vi "RTM - Export to XML.vi"(8 "error in (no error)":errorcluster, 11 "Node Ptr":u64 format="%.0x") -> (0 "error out":errorcluster)   [LabVIEW 2019, in "UDP-Custom-Device System Explorer.lvlib"]
uses:
  UDP-Custom-Device System Explorer.lvlib
panel:
  in  "Tag":string
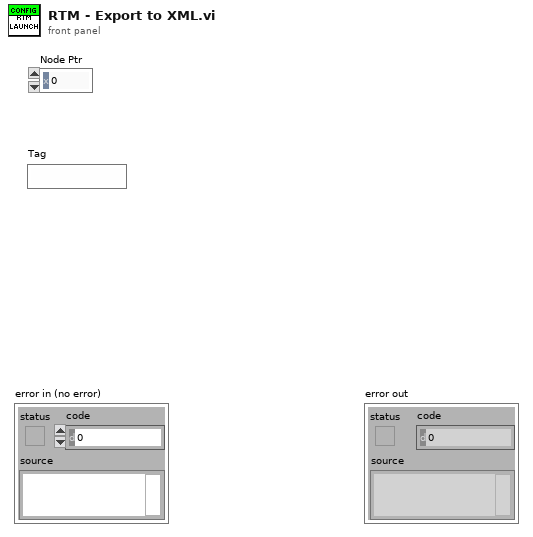
[diagram p1: front panel]
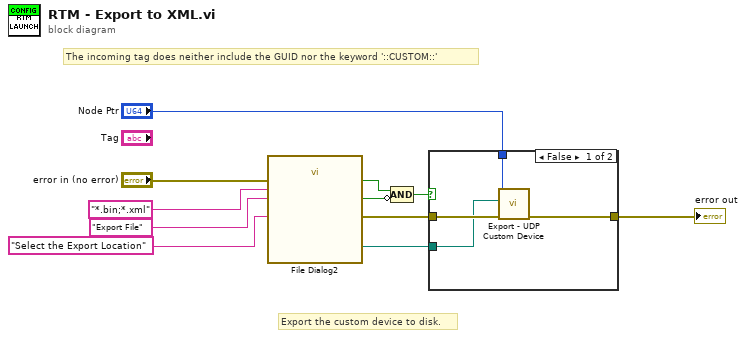
[diagram p0: block diagram]
diagram:
  # "Export the custom device to disk."
  # "The incoming tag does neither include the GUID nor the keyword '::CUSTOM::'"
  n1 = call "File Dialog2"("prompt"="Select the Export Location", "error in"="error in (no error)", "pattern (all files)"="*.bin;*.xml", "pattern label"="Export File") -> ("selected path"=w4:path, "exists"=w3:bool, "cancelled"=w2:bool, "error out"=w5:errorcluster)  [unwired: 8 in]
  n2 = Compound Arithmetic op=AND(w3, invert w2) -> (w1:bool)
  n3 = case shown="False" w1 {
    tunnel: "Node Ptr" -> [w15 _]
    tunnel: [w14 w16] -> w7
    tunnel: w5 -> [w13 w16]
    tunnel: w4 -> [w12 _]
    frame False {
      n4 = call "Export - UDP Custom Device.vi"("error in (no error)"=w13, "Target File"=w12, "Device Item Ref in"=w15) -> ("error out"=w14:errorcluster)  [unwired: 8 in]
    }
    frame True {
    }
  }
  "error out" <- w7
